vi "GetFilePath.vi"(8 "error in (no error)":errorcluster, 11 "DocumentClass in":refnum<class "Document.lvclass">) -> (0 "error out":errorcluster, 2 "FileName":path, 3 "DocumentClass out":refnum<class "Document.lvclass">)   [LabVIEW 2021, in "ProligentXMLGenerator.lvlib" / "Document.lvclass"]
doc: "The FileName is used to identify the type of document and should contain an extension so that the appropriate application is launched when the user requests to view the document content.\n\nLimited to 255 characters."
uses:
  Document.lvclass
  Document.lvclass/Document.ctl
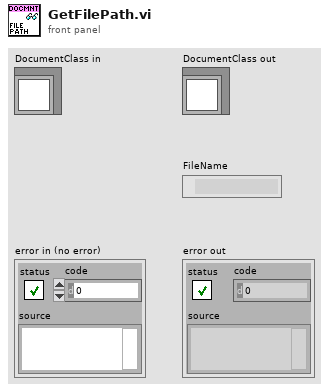
[diagram p1: front panel]
types:
  T1 = typedef "ProligentXMLGenerator.lvlib/Document.lvclass/Data.ctl" = cluster{"Name":string, "CustomData":refnum<class "CustomData.lvclass">, "Identifier":refnum<class "Guid.lvclass">, "NameType":refnum<class "NonEmptyString_255.lvclass">, "FileName":refnum<class "NonEmptyString_255.lvclass">, "Description":refnum<class "NonNullableString_600.lvclass">, "FilePath":path, "DestinationFolder":path}
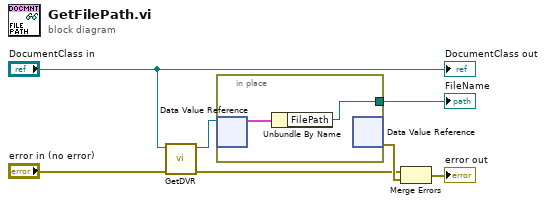
[diagram p0: block diagram]
diagram:
  n1 = call "GetDVR.vi"("error in"="error in (no error)", "Document in"="DocumentClass in") -> ("error out"=w2:errorcluster, "DVRReference"=w6:refnum<data-value>)  [unwired: 8 in]
  n2 = in-place "In Place Element Structure" {
    in-place-border: [w8] -> w1
    n3 = in-place-dvr #1(w6) -> (w9:T1)  [unwired: 1 out]
    n4 = Unbundle By Name(w9) -> ("FilePath"=w8:path)
    n5 = in-place-dvr #1() -> (w7:errorcluster)  [unwired: 1 in, 1 out]
  }
  "FileName" <- w1
  n6 = Merge Errors(w2, w7) -> (→"error out":errorcluster)
  "DocumentClass out" <- "DocumentClass in"
